vi "fgt trigger Ttl.vi"(8 "error in (no error)":errorcluster, 11 "TtlIndex":u32) -> (0 "error out":errorcluster)   [LabVIEW 2020, in "fgt_SDK.lvlib"]
doc: "Trigger a specific TTL port (BNC ports) if set as output."
uses:
  fgt_SDK.lvlib
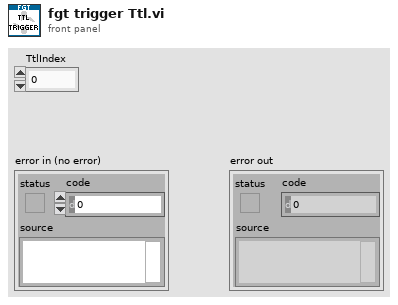
[diagram p1: front panel]
types:
  T1 = typedef "fgt_SDK.lvlib/fgt_STATUS_INFO.ctl" = cluster{"InstrType":T2, "instrSN":u16, "errorCode":u8, "infoCode":u8, "detail":string}
  T2 = typedef "fgt_SDK.lvlib/fgt_INSTRUMENT_TYPE.ctl" = enum32{"None", "MFCS", "MFCS_EZ", "FRP", "LineUP", "IPS"}
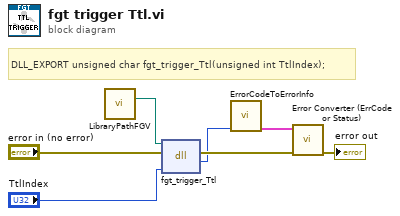
[diagram p0: block diagram]
diagram:
  # "DLL_EXPORT unsigned char fgt_trigger_Ttl(unsigned int TtlIndex);"
  n1 = call "LibraryPathFGV.vi"() -> ("Path Out"=w1:path)  [unwired: 14 in, 1 out]
  n2 = dll-call lib="C:/Workspace/fgt-SDK/LabVIEW/dlls/fgt_SDK_*.*" fn="fgt_trigger_Ttl"(path in=w1, error in="error in (no error)", "TtlIndex"="TtlIndex") -> (error out=w5:errorcluster, "return type"=w3:u8)  [unwired: 2 in, 1 out]
  n3 = call "ErrorCodeToErrorInfo.vi"("return type"=w3) -> ("StatusInfo"=w2:T1)  [unwired: 10 in]
  n4 = call "Error Converter (ErrCode or Status).vi"("error in (no error)"=w5, "StatusInfo"=w2) -> ("error out"=→"error out":errorcluster)  [unwired: 9 in]
